vi "Read Output Streams.vi"(8 "error in (no error)":errorcluster, 11 "ADAS PE Template Controller in":refnum<class "PE Controller.lvclass">) -> (0 "error out":errorcluster, 2 "Output Streams":T1[](array[typedef]), 3 "ADAS PE Template Controller out":refnum<class "PE Controller.lvclass">)   [LabVIEW 2020, in "ADAS PE Template.lvlib" / "PE Controller.lvclass"]
doc: "<b>Read Output Streams</b>\nThis VI lets PEF and the configuration utility know what the available output streams from this plugin are. The default is a single stream called \"Output\" - but many plugins will require multiple output streams. Further, to simplify configuration, it may make sense to rename the default output stream."
uses:
  PE Controller.lvclass
  <vilib>/FlexLogger/SDK/PluginSDK.lvlibp/PEFClasses/SDK/Processing Element Specification/Stream Specification.ctl
  <vilib>/FlexLogger/SDK/PluginSDK.lvlibp/PEFClasses/SDK/Processing Element Specification/Processing Element Specification.lvclass
panel:
  # "#via_ignore"
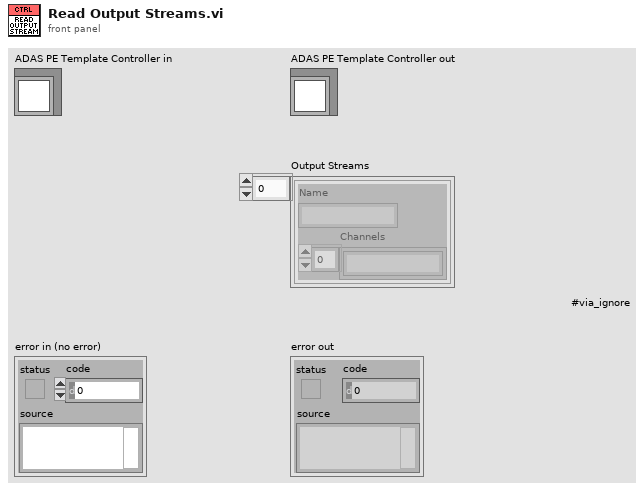
[diagram p1: front panel]
types:
  T1 = typedef "PluginSDK.lvlibp/Processing Element Specification.lvclass/Stream Specification.ctl" = cluster{"Name":string, "Channels":string[]}
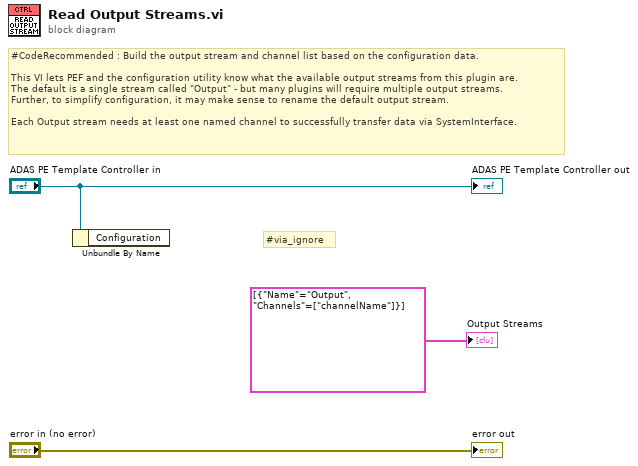
[diagram p0: block diagram]
diagram:
  # "#via_ignore"
  # "#CodeRecommended : Build the output stream and channel list based on the configuration data.\n\nThis VI lets PEF and the configuration utility know what the available output streams from this plugin are.\nThe default is a single stream called \"Output\" - but many plugins will require multiple output streams. \nFurther, to simplify configuration, it may make sense to rename the default output stream.\n\nEach Output stream needs at least one named channel to successfully transfer data via SystemInterface."
  n1 = Unbundle By Name("ADAS PE Template Controller in") -> ()  [unwired: 1 out]
  "error out" <- "error in (no error)"
  "ADAS PE Template Controller out" <- "ADAS PE Template Controller in"
  "Output Streams" <- T1[] [{"Name"="Output", "Channels"=["channelName"]}] ("Output Streams")
